vi "From 1D Path Tree Data.vi"(11 "Tree Data":refnum<class "Tree Data.lvclass">) -> (2 "1D Path":path[](array[path]))   [LabVIEW 2020, in "NI_VIAnCFGDataStructure.lvlib" / "1D Path.lvclass"]
doc: "Extract a 1D Path value from Tree Data type."
uses:
  <vilib>/addons/analyzer/VIAnCFGDataStructure/Data Types/Path Array/1D Path.lvclass
  <vilib>/addons/analyzer/VIAnCFGDataStructure/Tree Data/Tree Data.lvclass
  <vilib>/addons/analyzer/VIAnCFGDataStructure/Data Types/Path Array/1D Path.lvclass/1D Path.ctl
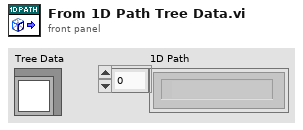
[diagram p1: front panel]
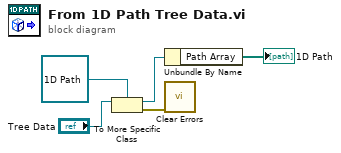
[diagram p0: block diagram]
diagram:
  n1 = To More Specific Class(target class=refnum<class "1D Path.lvclass"> refnum ("Path Array.lvclass"), reference="Tree Data") -> (specific class reference=w3:refnum<class "1D Path.lvclass">, error out=w2:errorcluster)  [unwired: 1 in]
  n2 = Unbundle By Name(w3) -> ("Path Array"=→"1D Path":path[])
  n3 = call <vilib>:"Clear Errors.vi"("error in (no error)"=w2) -> ()  [unwired: 5 in, 2 out]
